vi "displayFeedback.vi"(8 "error in (no error)":errorcluster, 10 "feedback_array":refnum<class "RobotFeedback.lvclass">[](array[class]), 11 "Communication in":refnum<class "Communication.lvclass">) -> (0 "error out":errorcluster, 1 "robotDisplayFeedback":T1[](array[typedef]) {"Battery (V)" scale=6.0..8.4}, 2 "feedback_array out":refnum<class "RobotFeedback.lvclass">[](array[class]), 3 "Communication out":refnum<class "Communication.lvclass">)   [LabVIEW 2021, in "Communication.lvclass"]
uses:
  Communication.lvclass
  RobotFeedback/RobotFeedback.lvclass
  Robot_class/robotDisplayFeedback.ctl
  <vilib>/wsapi/NI_WebServices.lvlib
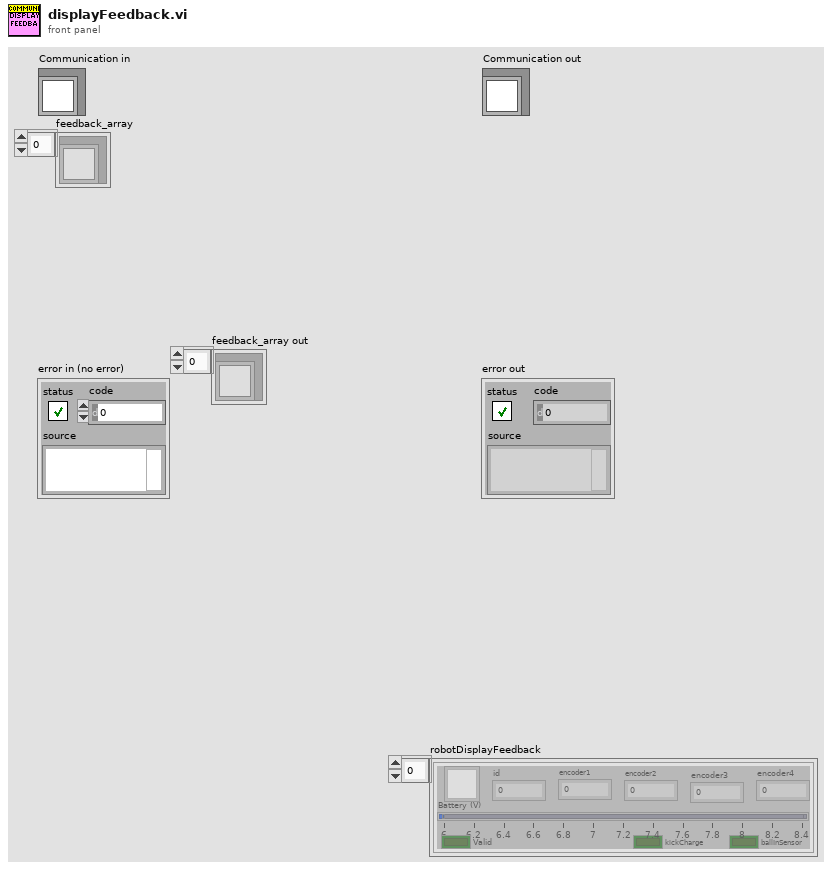
[diagram p1: front panel]
types:
  T1 = typedef "robotDisplayFeedback.ctl" = cluster{"id":dbl, "encoder1":dbl, "encoder2":dbl, "kickCharge":bool, "ballInSensor":bool, "Battery (V)":dbl, "2D Picture":picture, "encoder3":dbl, "encoder4":dbl, "Valid":bool}
  T2 = typedef "imagedata.ctl" = cluster{"image type":i32, "image depth":i32, "image":u8[], "mask":u8[], "colors":u32[], "Rectangle":cluster{"left":i16, "top":i16, "right":i16, "bottom":i16}}
  T3 = typedef "feedbackData.ctl" = cluster{"id":u32, "status":u32, "battery":sgl, "encoder1":sgl, "encoder2":sgl, "encoder3":sgl, "encoder4":sgl}
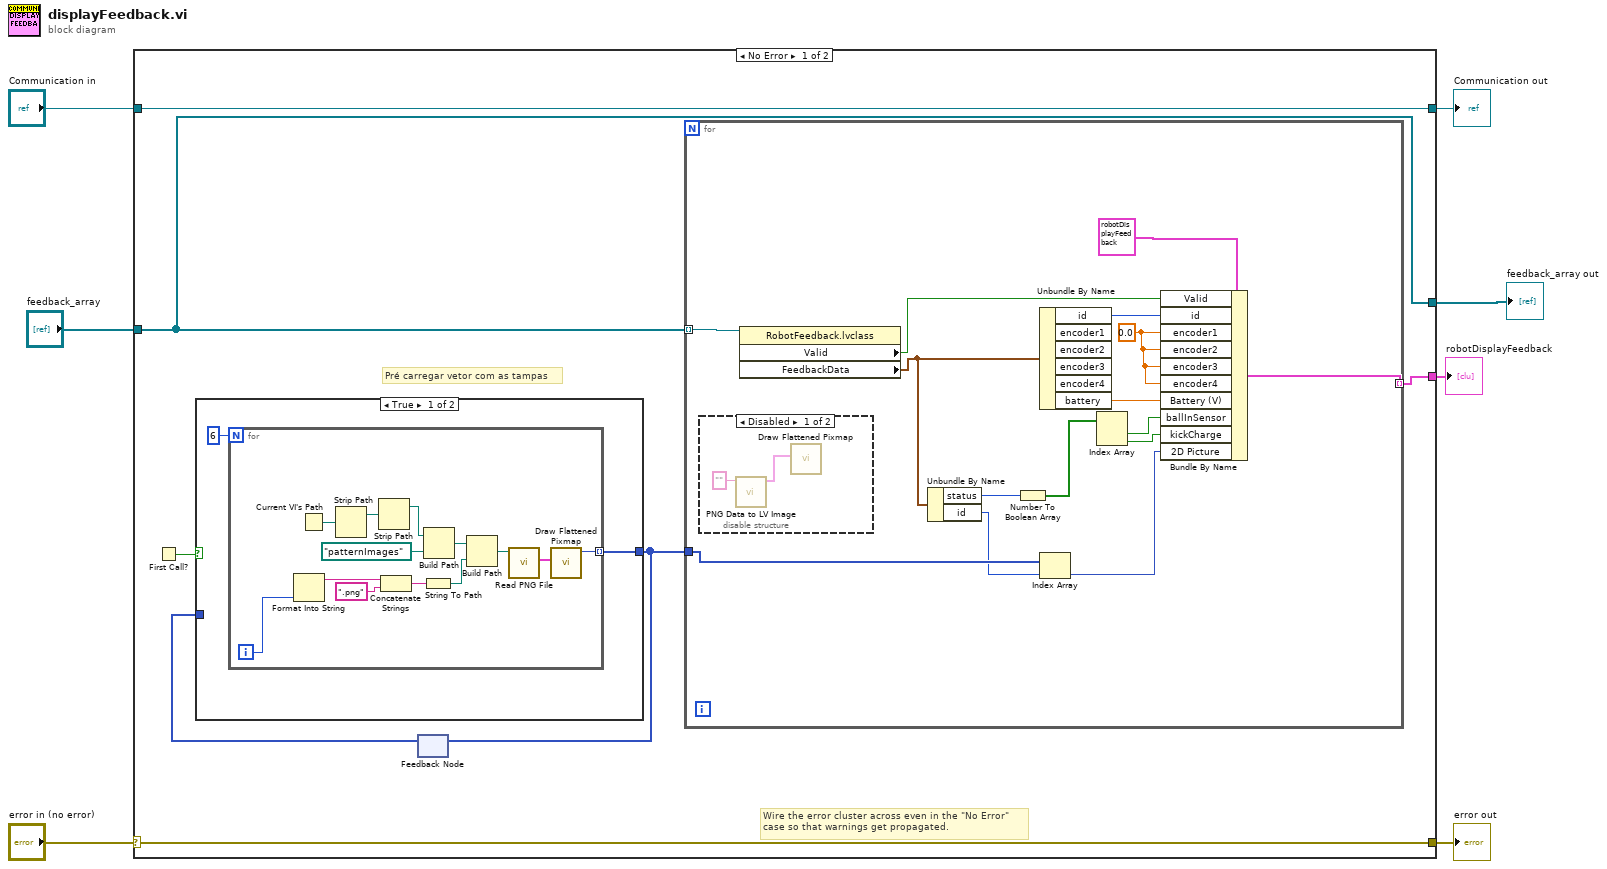
[diagram p0: block diagram]
diagram:
  n1 = case shown="No Error" "error in (no error)" {
    selector: "error in (no error)" -> [w13 w49]
    tunnel: [w13 w49] -> w6
    tunnel: [w14 w48] -> w4
    tunnel: "Communication in" -> [w14 w48]
    tunnel: "feedback_array" -> [w11 _]
    tunnel: [w12 _] -> w1
    tunnel: [w11 _] -> w2
    frame No Error {
      # "Pré carregar vetor com as tampas"
      # "Wire the error cluster across even in the \"No Error\"\ncase so that warnings get propagated."
      n2 = First Call?() -> (First Call?: T/F=w10:bool)
      n3 = feedback #1() -> (w9:picture[])  [unwired: 1 in]
      n4 = case shown="True" w10 {
        tunnel: [w15 w30] -> w8
        tunnel: w9 -> [_ w30]
        frame True {
          n5 = for {
            N: 6 -> [_]
            tunnel: [w17] -> w15 mode=indexing
            i -> [w18]
            n6 = Format Into String(w18) -> (resulting string=w22:string)  [unwired: 3 in, 1 out]
            n7 = Current VI's Path() -> (path=w25:path)
            n8 = Strip Path(path=w25) -> (stripped path=w26:path)  [unwired: 1 out]
            n9 = Strip Path(path=w26) -> (stripped path=w27:path)  [unwired: 1 out]
            n10 = Concatenate Strings(w22, ".png" ("string")) -> (w20:string)
            n11 = String To Path(string=w20) -> (path=w19:path)
            n12 = Build Path(base path=w27, name or relative path=path "patternImages") -> (appended path=w28:path)
            n13 = Build Path(base path=w28, name or relative path=w19) -> (appended path=w29:path)
            n14 = call <vilib>:"Read PNG File.vi"("path to PNG file"=w29) -> ("image data"=w23:T2)  [unwired: 8 in, 2 out]
            n15 = call <vilib>:"Draw Flattened Pixmap.vi"("image data"=w23) -> ("new picture"=w17:picture)  [unwired: 8 in]
          }
        }
        frame False {
        }
      }
      n16 = feedback-in #1(w8) -> ()
      n17 = for {
        tunnel: w11 -> [w45] mode=indexing
        tunnel: [w37] -> w12 mode=indexing
        tunnel: w8 -> [w34]
        w31 = 0.0 ("encoder1")
        n18 = disable-structure shown="Disabled" {
          frame Disabled {
            n19 = call <vilib>:"PNG Data to LV Image.vi"("png data"="") -> ("image data"=w46:T2)  [unwired: 9 in, 1 out]
            n20 = call <vilib>:"Draw Flattened Pixmap.vi"("image data"=w46) -> ()  [unwired: 8 in, 1 out]
          }
          frame Enabled {
          }
        }
        n21 = property class="RobotFeedback.lvclass"(reference=w45) -> ("Valid"=w35:bool, "FeedbackData"=w42:T3)  [unwired: 1 in, 2 out]
        n22 = Unbundle By Name(w42) -> ("status"=w41:u32, "id"=w33:u32)
        n23 = Number To Boolean Array(number=w41) -> (Boolean array=w40:bool[])
        n24 = Unbundle By Name(w42) -> ("id"=w44:u32, "battery"=w43:sgl)  [unwired: 4 out]
        n25 = Index Array(array=w34, index=w33) -> (element=w32:picture)
        n26 = Index Array(array=w40) -> (element #1=w39:bool, element #2=w38:bool)  [unwired: 2 in]
        n27 = Bundle By Name(cluster=T1 {"id"=0.0, "encoder1"=0.0, "encoder2"=0.0, "kickCharge"=FALSE, "ballInSensor"=FALSE, "Battery (V)"=0.0, "2D Picture"=bytes[0], "encoder3"=0.0, "encoder4"=0.0, "Valid"=FALSE} ("RobotDisplayFeedback"), "Valid"=w35, "id"=w44, "encoder1"=w31, "encoder2"=w31, "encoder3"=w31, "encoder4"=w31, "Battery (V)"=w43, "ballInSensor"=w39, "kickCharge"=w38, "2D Picture"=w32) -> (w37:T1)
      }
    }
    frame Error {
    }
  }
  "error out" <- w6
  "Communication out" <- w4
  "feedback_array out" <- w2
  "robotDisplayFeedback" <- w1
